vi "DAQmx Clear Task.vi"(0 "task in":refnum<k21>, 11 "error in":errorcluster) -> (15 "error out":errorcluster)   [LabVIEW 2017]
doc: "Clears the task. Before clearing, this VI aborts the task, if necessary, and releases any resources the task reserved. You cannot use a task after you clear it unless you recreate the task."
uses:
  nilvaiu.dll
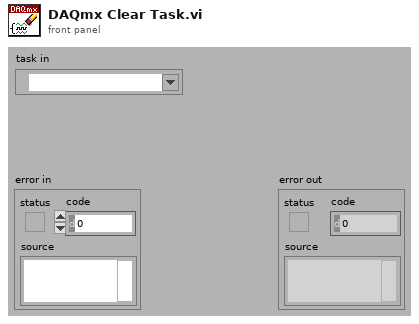
[diagram p1: front panel]
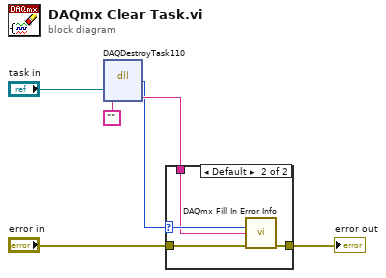
[diagram p0: block diagram]
diagram:
  n1 = dll-call lib="nilvaiu.*" fn="DAQDestroyTask110"("taskRefObjPtr"="task in", "errorInfo"="") -> (w4:i32, "errorInfo"=w6:string)  [unwired: 4 in, 2 out]
  n2 = case shown="Default" w4 {
    selector: w4 -> [_ w9]
    tunnel: "error in" -> [w7 w11]
    tunnel: [w7 w10] -> w5
    tunnel: w6 -> [_ w8]
    frame 0 {
    }
    frame Default {
      n3 = call "DAQmx Fill In Error Info.vi"("status code"=w9, "extended error info"=w8, "error in"=w11) -> ("error out"=w10:errorcluster)  [unwired: 1 in, 11 out]
    }
  }
  "error out" <- w5
